vi "RTS Cool Dehum Calcs.vi"(11 "Chamber 1-3":T1[](array[typedef]) {"Start Time" format="%<%X\n%x>T"; "End Time" format="%<%X\n%x>T"}) -> (3 "Array":T1[](array[typedef]) {"Start Time" format="%<%X\n%x>T"; "End Time" format="%<%X\n%x>T"})   [LabVIEW 2020]
uses:
  Type Definitions/RTS Door Ops Client.ctl
  Type Definitions/RTS Door Opening Schedule.ctl
  Type Definitions/RTS Door Ops Sequence.ctl
  Type Definitions/RTS Chamber Temperature Humidity Control.ctl
panel:
  out "Error Out":errorcluster
  in  "Error In":errorcluster
  # "Chamber Conditions:"
  # "Chamber Conditions:"
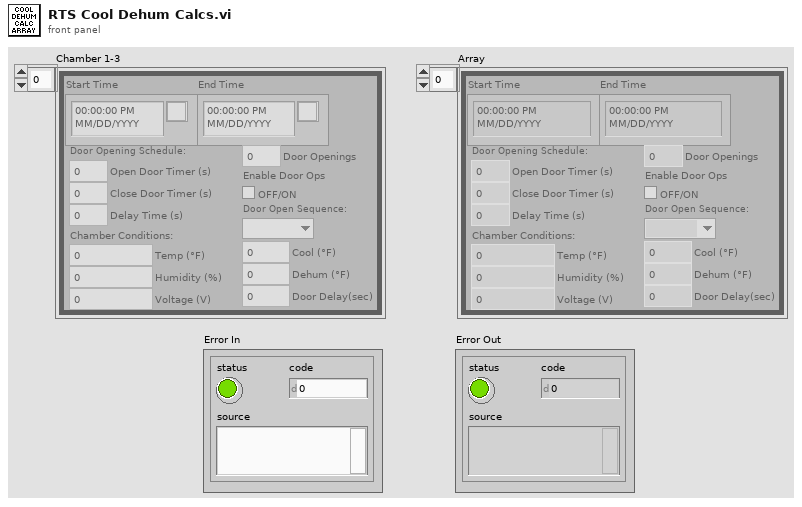
[diagram p1: front panel]
types:
  T1 = typedef "RTS Door Ops Client.ctl" = cluster{"End Time":timestamp, "Start Time":timestamp, "Door Opening Schedule:":T2, "Enable Door Ops":bool, "Door Openings":u32, "Temp (°F)":dbl, "Humidity (%)":dbl, "Voltage (V)":dbl, "Door Open Sequence:":T3, "Door Delay(sec)":dbl, "Dehum (°F)":dbl, "Cool (°F)":dbl}
  T2 = typedef "RTS Door Opening Schedule.ctl" = cluster{"Open Door Timer (s)":dbl, "Delay Time (s)":dbl, "Close Door Timer (s)":dbl}
  T3 = typedef "RTS Door Ops Sequence.ctl" = enum16{"", "1st", "2nd", "3rd"}
  T4 = typedef "RTS Chamber Temperature Humidity Control.ctl" = cluster{"Room Setpoint Temperature (*RM Dry Set P1)":dbl, "Room Setpoint Humidity (*RM Hum Set P1)":dbl, "Room Cool Temperature (*RM Cool Setp 1)":dbl, "Room Dehum Temperature (*RM De Hum Set P1)":dbl}
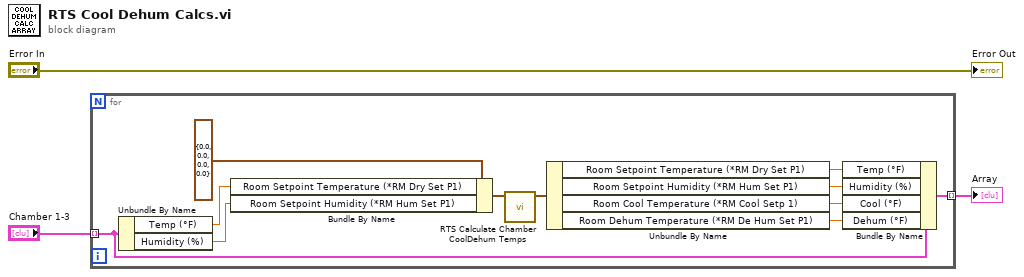
[diagram p0: block diagram]
diagram:
  n1 = for {
    tunnel: "Chamber 1-3" -> [w10] mode=indexing
    tunnel: [w4] -> w3 mode=indexing
    n2 = Unbundle By Name(w10) -> ("Temp (°F)"=w14:dbl, "Humidity (%)"=w13:dbl)
    n3 = Bundle By Name(cluster=T4 {"Room Setpoint Temperature (*RM Dry Set P1)"=0.0, "Room Setpoint Humidity (*RM Hum Set P1)"=0.0, "Room Cool Temperature (*RM Cool Setp 1)"=0.0, "Room Dehum Temperature (*RM De Hum Set P1)"=0.0} ("Room Setpoints"), "Room Setpoint Temperature (*RM Dry Set P1)"=w14, "Room Setpoint Humidity (*RM Hum Set P1)"=w13) -> (w12:T4)
    n4 = call "RTS Calculate Chamber CoolDehum Temps.vi"("Room Setpoints"=w12) -> ("Room Setpoint Output"=w9:T4)  [unwired: 9 in, 1 out]
    n5 = Unbundle By Name(w9) -> ("Room Setpoint Temperature (*RM Dry Set P1)"=w8:dbl, "Room Setpoint Humidity (*RM Hum Set P1)"=w7:dbl, "Room Cool Temperature (*RM Cool Setp 1)"=w6:dbl, "Room Dehum Temperature (*RM De Hum Set P1)"=w5:dbl)
    n6 = Bundle By Name(cluster=w10, "Temp (°F)"=w8, "Humidity (%)"=w7, "Cool (°F)"=w6, "Dehum (°F)"=w5) -> (w4:T1)
  }
  "Array" <- w3
  "Error Out" <- "Error In"
